vi "get_SampleHandler_state_cleanup.vi"(8 "error in (no error)":errorcluster caption="エラー入力（エラーなし）", 11 "VISAリソース名":refnum<visa-resource-name>) -> (0 "error out":errorcluster caption="エラー出力", 3 "VISAリソース名（出力）":refnum<visa-resource-name>)   [LabVIEW 2017]
panel:
  out "数値":dbl
  out "文字列":string
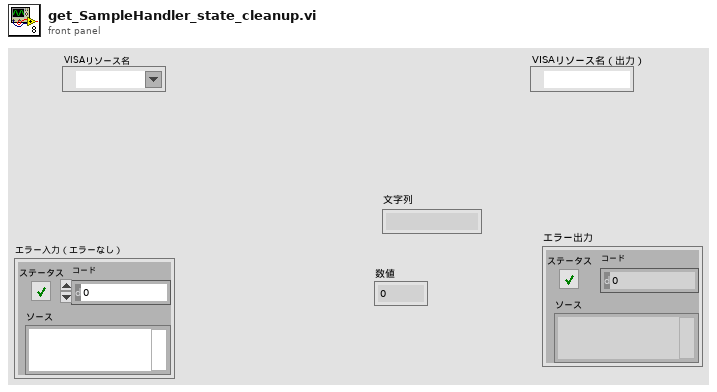
[diagram p1: front panel]
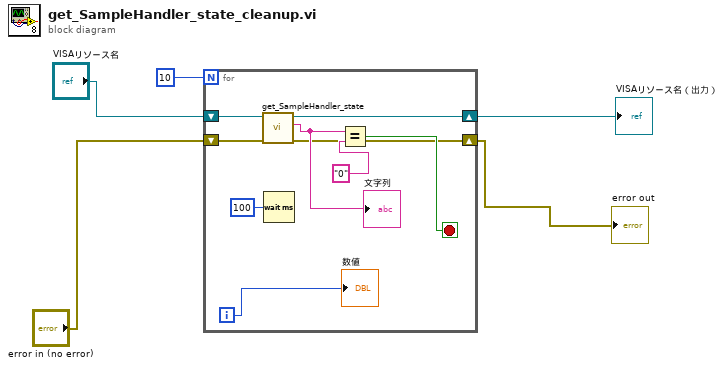
[diagram p0: block diagram]
diagram:
  n1 = for {
    N: 10 -> [_]
    shift-right: [w9] -> w3
    shift-left: "VISAリソース名" -> [w14]
    shift-right: [w7] -> w1
    shift-left: "error in (no error)" -> [w13]
    i -> [w6]
    stop <- w10 stop-if-true
    n2 = call "get_SampleHandler_state.vi"("error in (no error)"=w13, "VISAリソース名"=w14) -> ("error out"=w7:errorcluster, "response"=w8:string, "VISAリソース名（出力）"=w9:refnum<visa-resource-name>)  [unwired: 7 in]
    "文字列" <- w8
    n3 = Wait (ms)(milliseconds to wait=100) -> ()  [unwired: 1 out]
    n4 = Equal?(x=w8, y="0") -> (x = y?=w10:bool)
    "数値" <- w6
  }
  "VISAリソース名（出力）" <- w3
  "error out" <- w1
